vi "CurrentCollectOnly.vi"() -> ()   [LabVIEW 2018]
uses:
  <vilib>/Utility/file.llb/Write Delimited Spreadsheet (string).vi
  Drivers/Agilent 34972/Agilent 34970.lvlib
panel:
  in  "Agilent Scan Rate (Seconds)":i32=3
  in  "Start DAQ Loop":bool
  out "Collecting Agilent Data":bool
  in  "Lab?":string="Washer HCC"
  in  "?":enum32{"Main", "Extra", "Debug"}(tab)
  in  "34972-1":refnum<visa-resource-name>="AGILENT_HCC"
  in  "error in (no error)":errorcluster
  out "error out":errorcluster
  out "Data Folder":path
  out "Current Data (for each station)":string[][](array[string])
  out "XY Graph":T1(graph)
  in  "X-Axis":string(combo)
  in  "Y-Axis-1":string(combo)
  in  "Y-Axis-2":string(combo)
  out "Agilent Channels DAQ":string
  out "read buffer":string
  in  "Status Output Locations":path[](array[path])
  in  "Connected Board ID's (Newfi)":string[](array[string])
  in  "Total Array":string[][](array[string])
  out "Main Loop Rate":dbl format="%0.2f"
  out "Station IDs":string[](array[string])=["2M1", "2M2", "2M3", "2M4", "2M5", "2M6", "2M7", "2M8", "2M9", "2M10", "2M11", "2M12", "2M13", "2M14", "2M15", "2M16", "2M17", "2M18", "2M19", "2M20", "N/A", "N/A", "N/A", "N/A"]
  in  "file path (use dialog)":path
  out "DAQ Loop":string[](array[string])
  in  "Debug":bool
  in  "Timer":dbl format="%<%H:%M:%S>t"
  in  "QUIT":bool
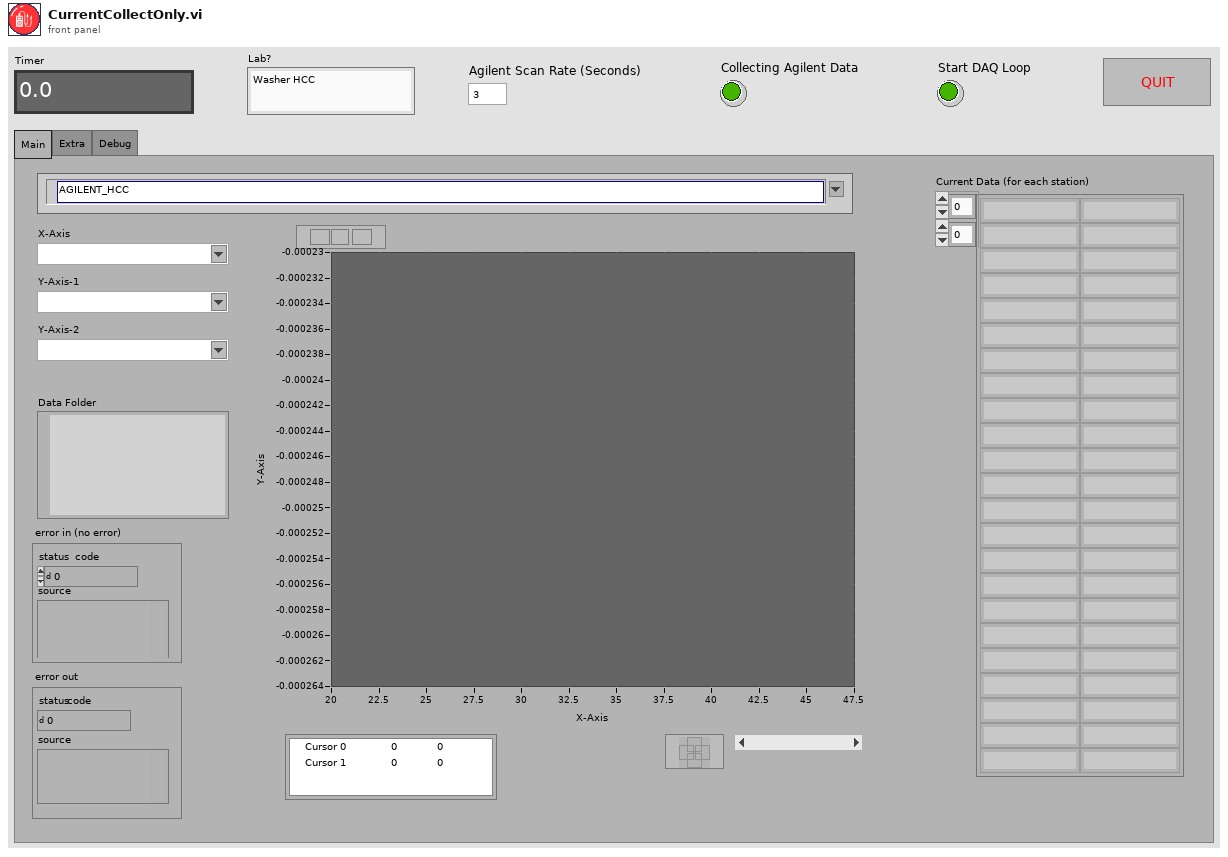
[diagram p1: front panel]
types:
  T1 = cluster{"Time Array Output":dbl[], "Data Array Output":dbl[]}[]
  T2 = cluster{"34972-1":refnum<visa-resource-name>, "Agilent Scan Rate (Seconds)":i32, "Current":dbl[], "Voltage":dbl[], "Agilent Channels DAQ":string, "file path (use dialog)":path, "Timer":dbl, "Total Array":string[][], "Station IDs":string[], "Connected Board ID's (Newfi)":string[], "Status Output Locations":path[], "Lab?":string, "Plot Array":dbl[][]}
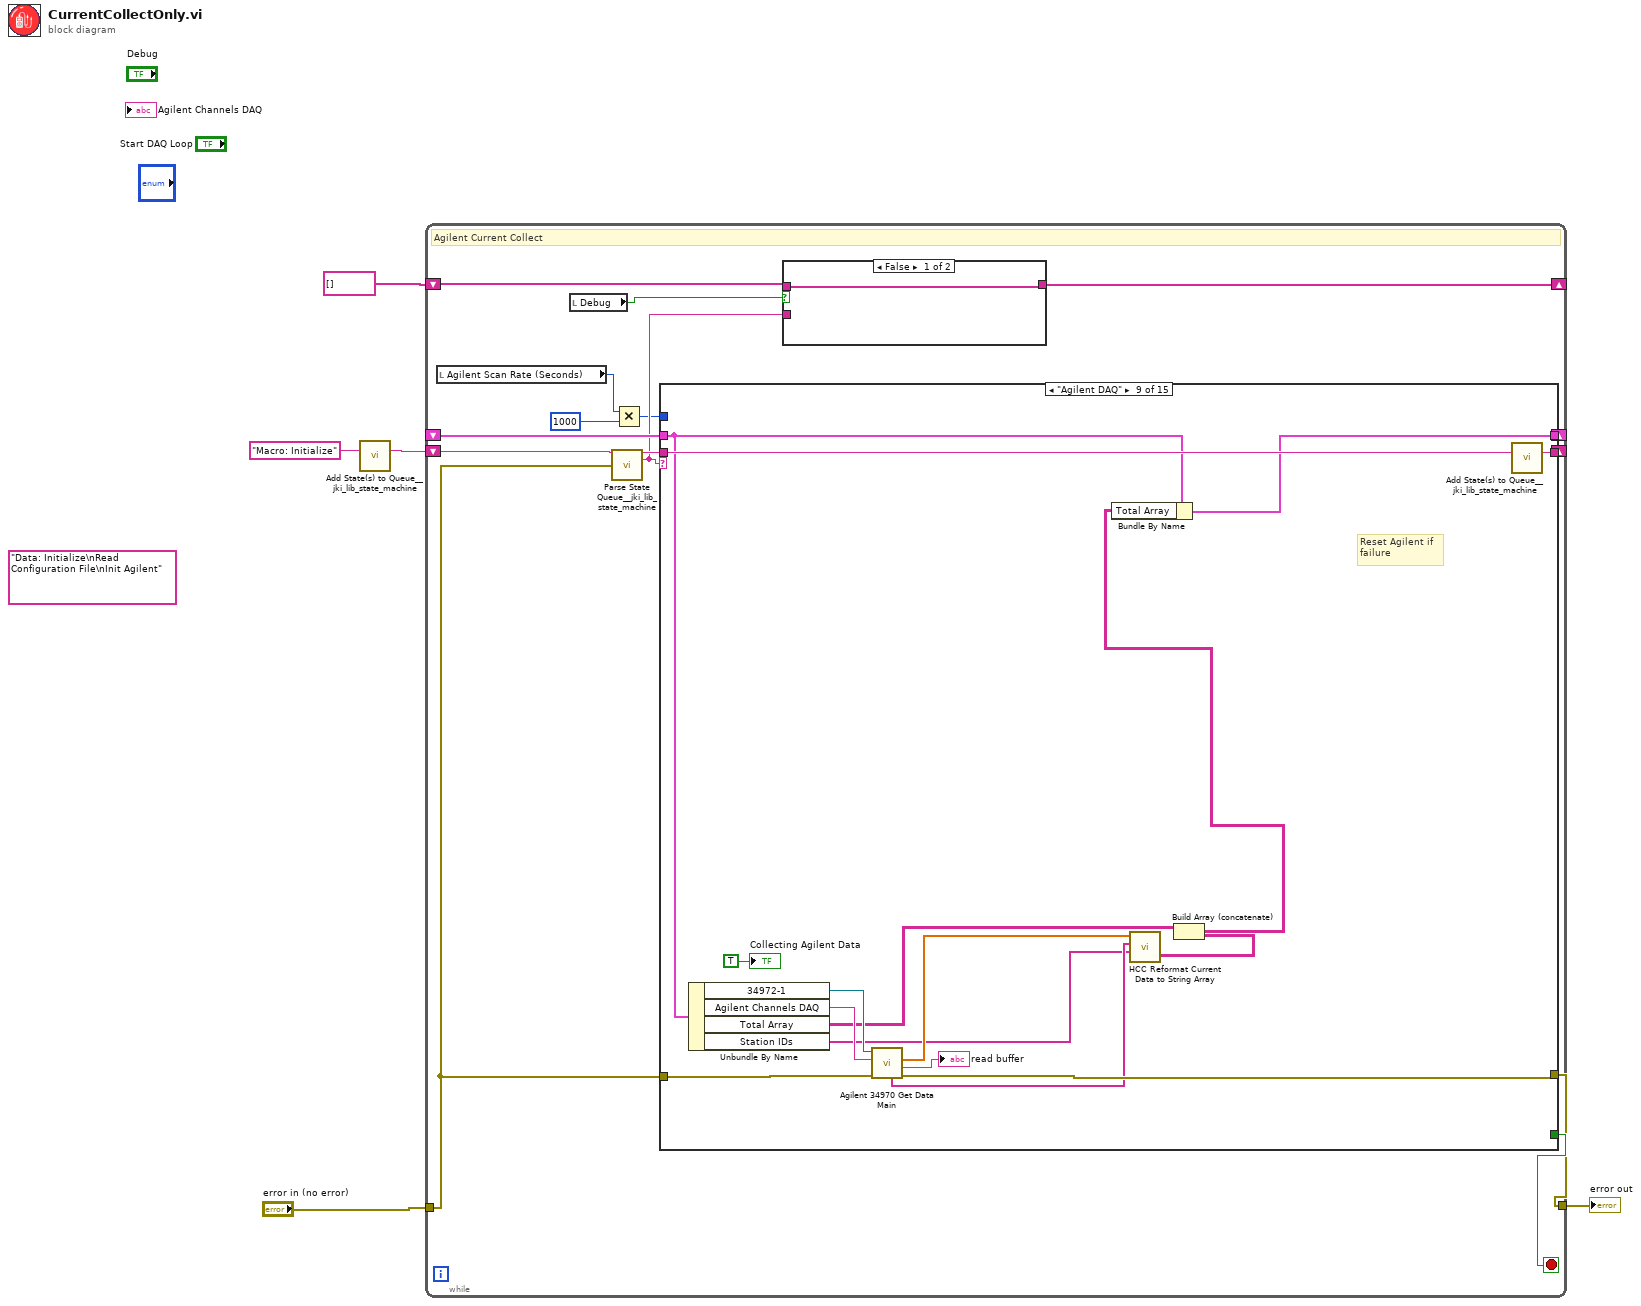
[diagram p0: block diagram]
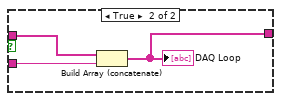
[diagram p2: hidden frame]
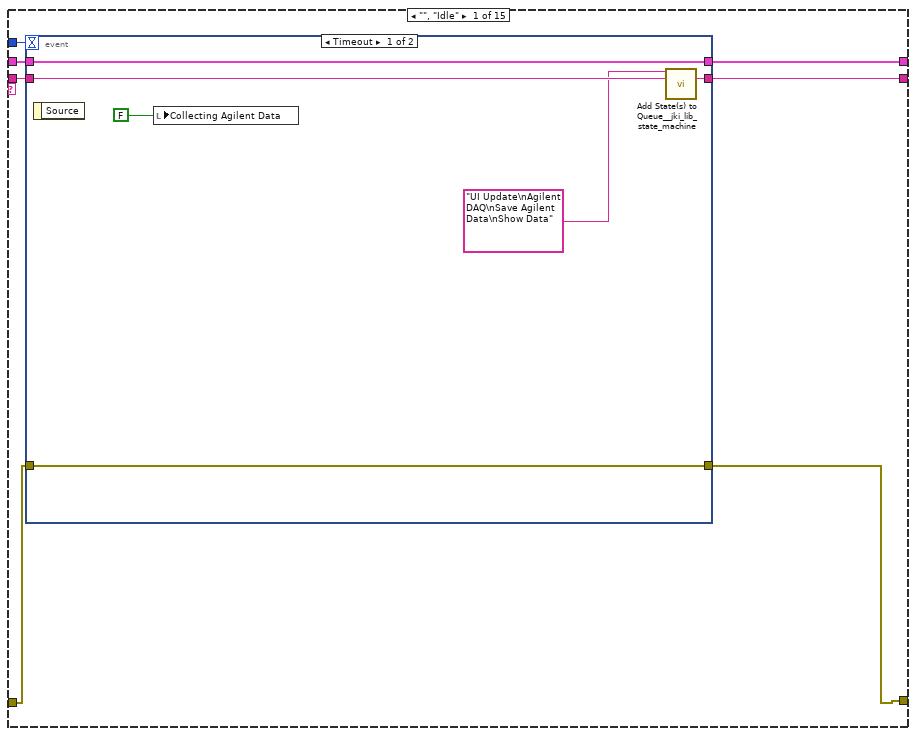
[diagram p3: hidden frame]
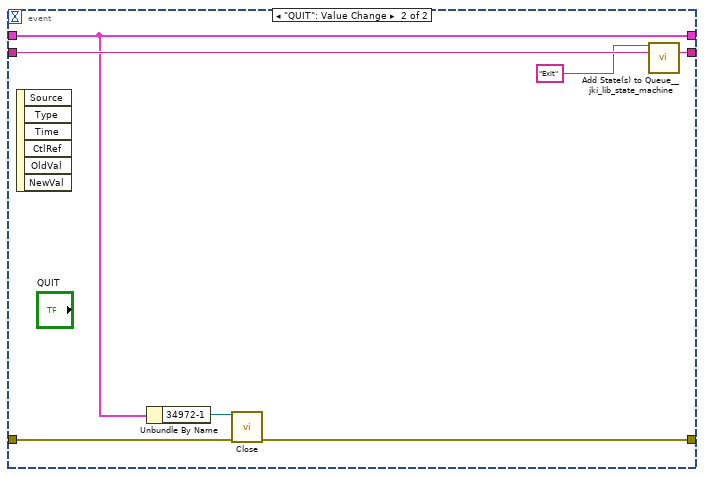
[diagram p4: hidden frame]
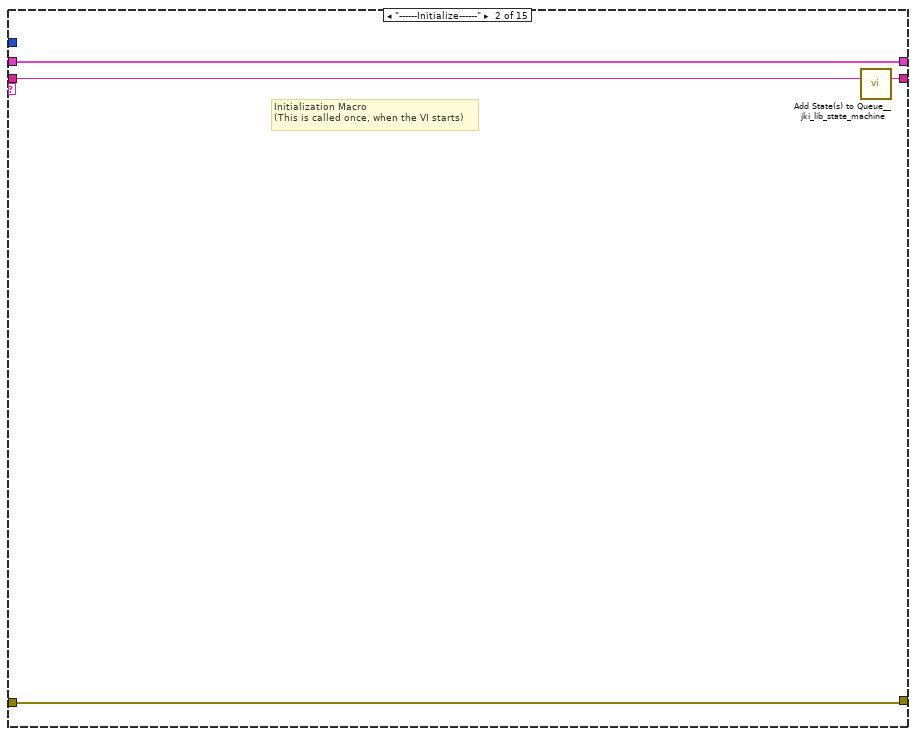
[diagram p5: hidden frame]
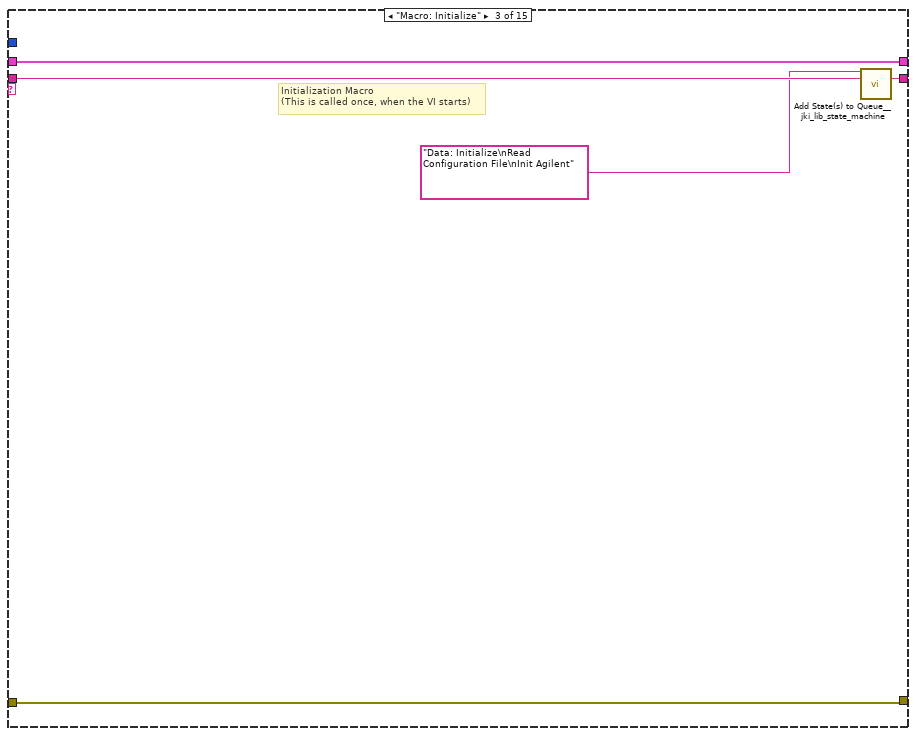
[diagram p6: hidden frame]
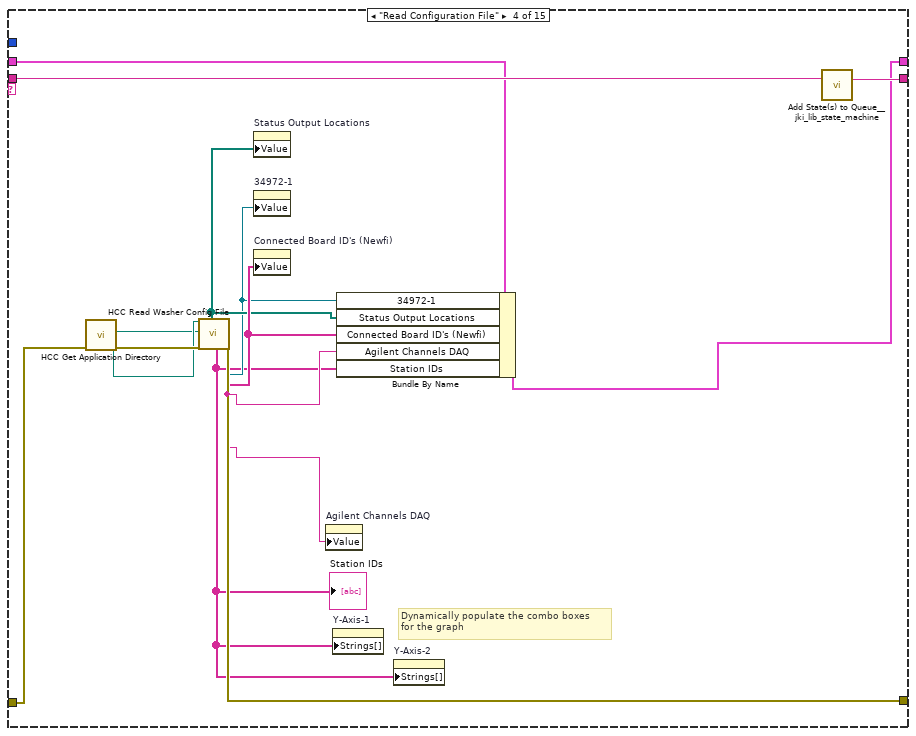
[diagram p7: hidden frame]
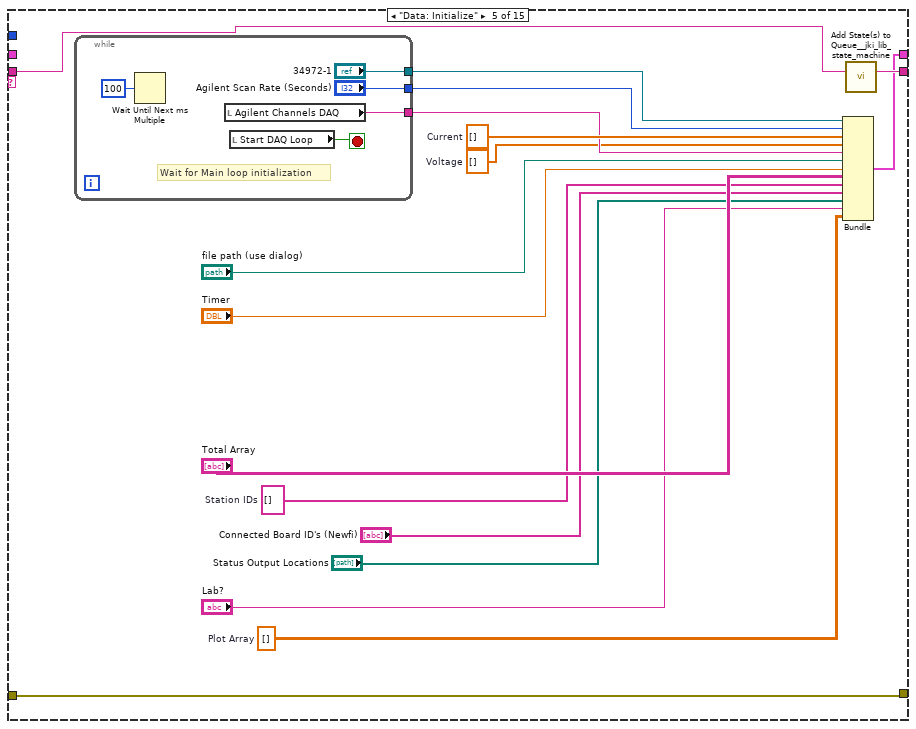
[diagram p8: hidden frame]
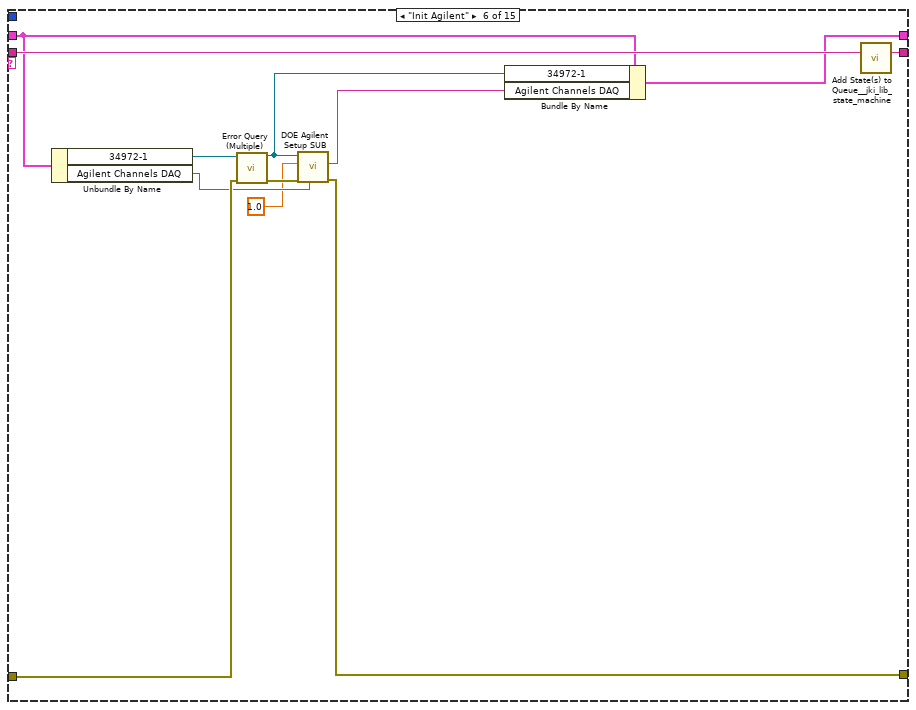
[diagram p9: hidden frame]
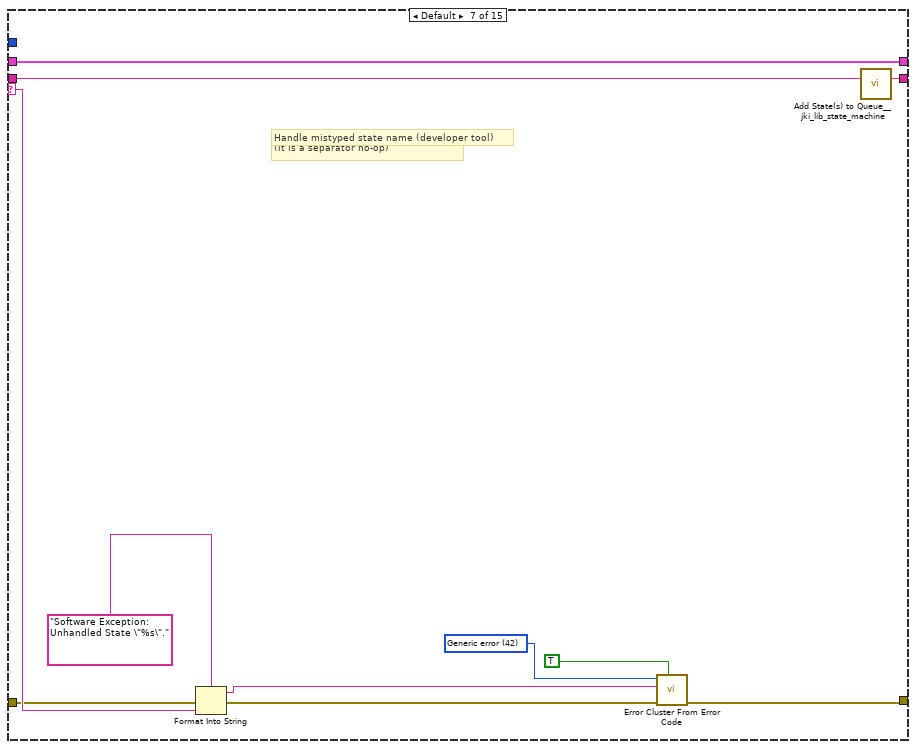
[diagram p10: hidden frame]
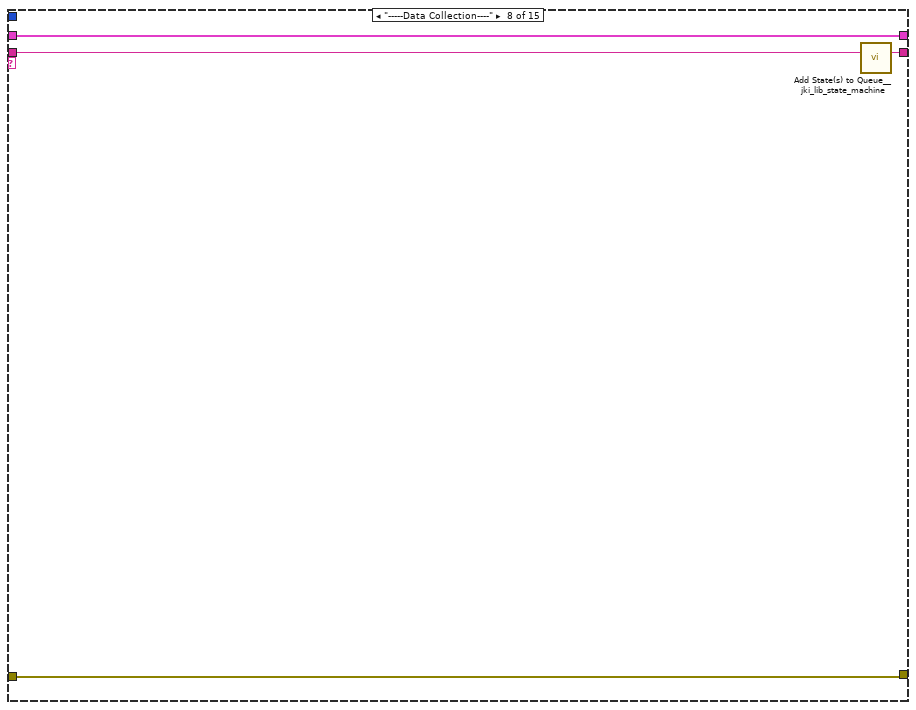
[diagram p11: hidden frame]
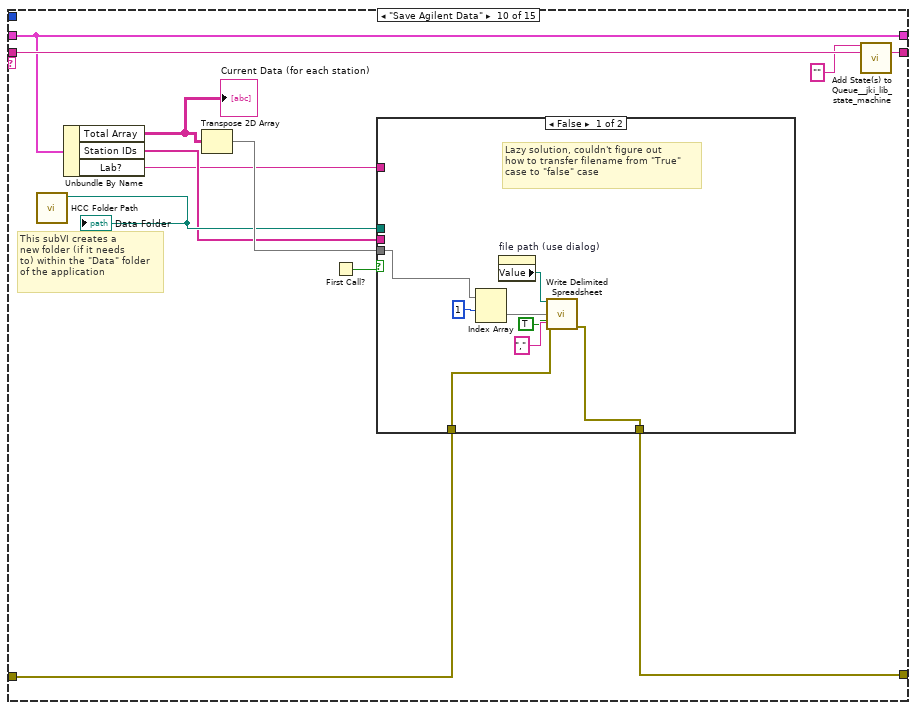
[diagram p12: hidden frame]
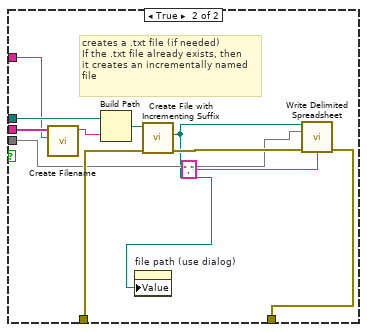
[diagram p13: hidden frame]
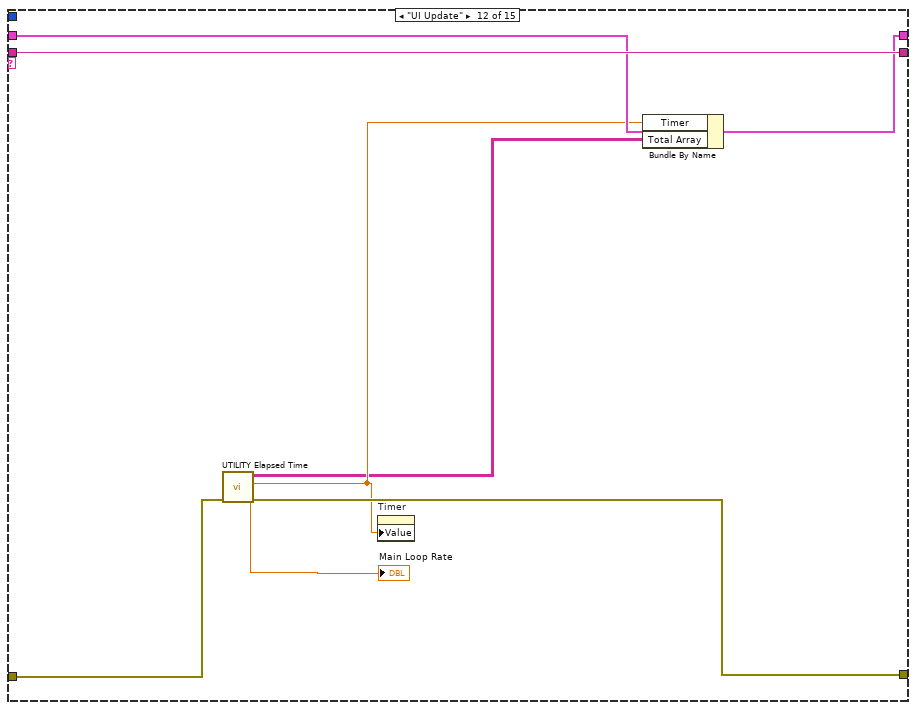
[diagram p15: hidden frame]
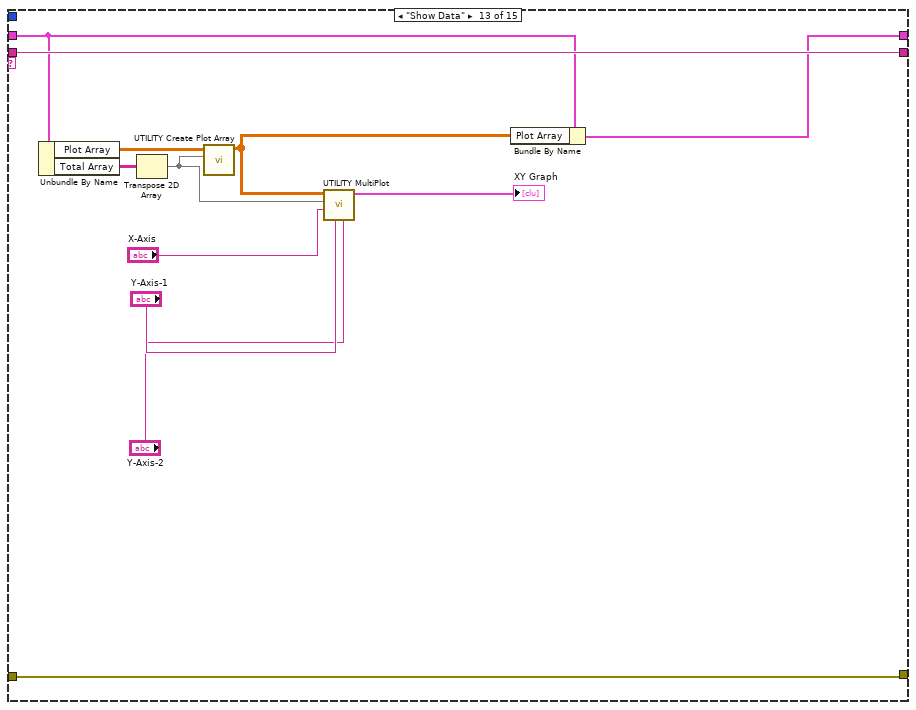
[diagram p16: hidden frame]
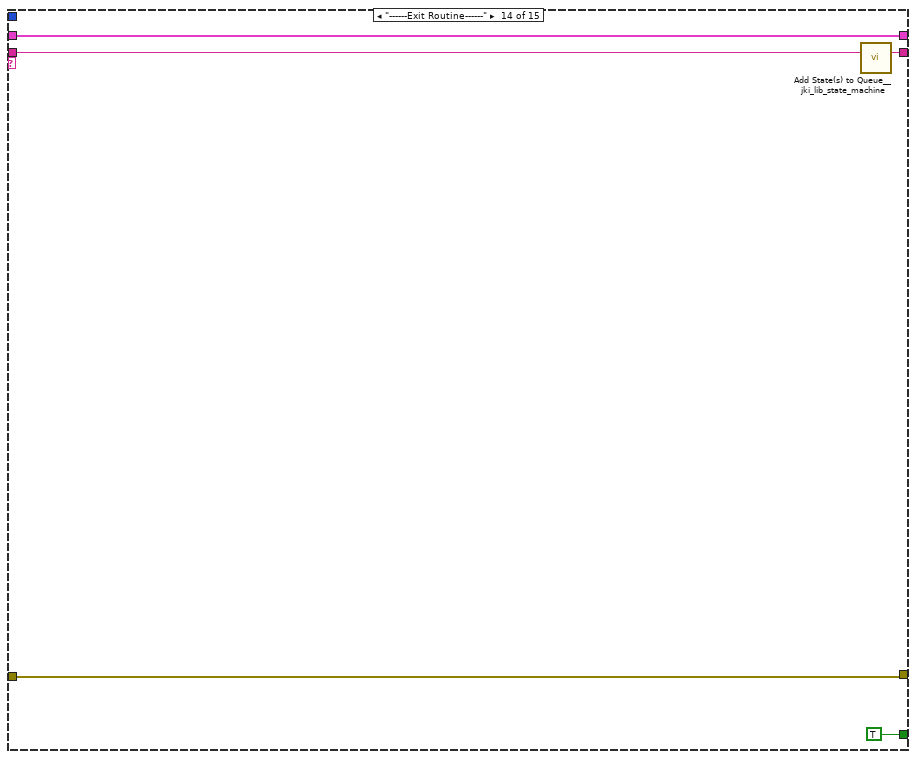
[diagram p17: hidden frame]
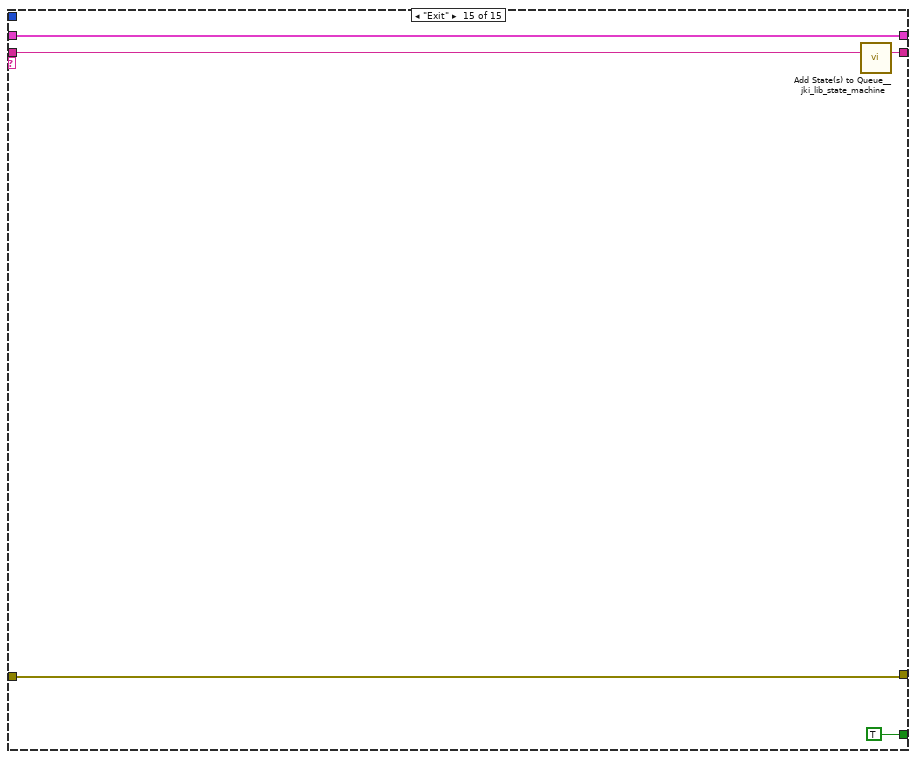
[diagram p18: hidden frame]
diagram:
  (unwired) "Data: Initialize\nRead Configuration File\nInit Agilent"
  n1 = call <vilib>:"Add State(s) to Queue__jki_lib_state_machine.vi"("State(s) in (\"\")"="Macro: Initialize") -> ("States Out"=w3:string)  [unwired: 14 in]
  n2 = while "Agilent DAQ and Save" {
    shift-right: [w6] -> _
    shift-left: _ -> [w17]
    shift-right: [w7] -> _
    shift-left: w3 -> [w19]
    tunnel: "error in (no error)" -> [w15]
    tunnel: [w16] -> w5
    shift-right: [w12] -> _
    shift-left: string[] [] -> [w14]
    stop <- w18 stop-if-true
    # "Agilent Current Collect"
    n3 = local read "Agilent Scan Rate (Seconds)"() -> (w10:i32)
    n4 = local read "Debug"() -> (w11:bool)
    n5 = call <vilib>:"Parse State Queue__jki_lib_state_machine.vi"("State Queue"=w19, "Error In (no error)"=w15) -> ("Remaining States"=w20:string, "Current State"=w13:string)  [unwired: 11 in, 1 out]
    n6 = Multiply(x=w10, y=1000) -> (x*y=w8:i32)
    n7 = case shown="\"Agilent DAQ\"" w13 {
      selector: w13 -> [_ _ _ _ _ _ w104 _ _ _ _ _ _ _ _]
      tunnel: w20 -> [w31 w48 w53 w62 w75 w101 w112 w116 w132 w144 w165 w173 w185 w191 w196]
      tunnel: w17 -> [w29 w46 w51 w61 _ w99 w110 w114 w121 w141 w166 w169 w177 w189 w194]
      tunnel: [_ _ _ _ _ _ _ _ _ _ _ _ _ TRUE TRUE] -> w18
      tunnel: w8 -> [w27 _ _ _ _ _ _ _ _ _ _ _ _ _ _]
      tunnel: w15 -> [w26 w45 w49 w67 w81 w96 w103 w113 w129 w139 w164 w174 w186 w187 w192]
      tunnel: [w25 w45 w49 w65 w81 w90 w102 w113 w125 w138 w164 w171 w186 w187 w192] -> w16
      tunnel: [w30 w47 w52 w63 w84 w100 w111 w115 w131 w143 w165 w173 w185 w190 w195] -> w7
      tunnel: [w28 w46 w51 w58 w83 w98 w110 w114 w119 w141 w166 w170 w175 w189 w194] -> w6
      frame "", "Idle" {
        n8 = event shown="[0] Timeout" {
          selector: _ -> [_ _]
          dyn-events: _ -> [_ _]
          timeout: w27 -> [_ _]
          tunnel: w31 -> [w37 w44]
          tunnel: [w36 w43] -> w30
          tunnel: w29 -> [w35 w41]
          tunnel: [w35 w41] -> w28
          tunnel: [w32 w38] -> w25
          tunnel: w26 -> [w32 w39]
          event Timeout {
            n9 = event-data() -> ()  [unwired: 1 in, 1 out]
            n10 = local write "Collecting Agilent Data"(FALSE ("Collecting Agilent Data")) -> ()
            n11 = call <vilib>:"Add State(s) to Queue__jki_lib_state_machine.vi"("State(s) in Front (\"\")"="UI Update\nAgilent DAQ\nSave Agilent Data\nShow Data", "State(s) in (\"\")"=w37) -> ("States Out"=w36:string)  [unwired: 13 in]
          }
          event "QUIT": Value Change {
            n12 = event-data() -> ()  [unwired: 1 in, 6 out]
            n13 = Unbundle By Name(w41) -> ("34972-1"=w40:refnum<visa-resource-name>)
            n14 = call "Close.vi"("VISA Resource Name"=w40, "error in (no error)"=w39) -> ("error out"=w38:errorcluster)  [unwired: 13 in]
            n15 = call <vilib>:"Add State(s) to Queue__jki_lib_state_machine.vi"("State(s) in Front (\"\")"="Exit", "State(s) in (\"\")"=w44) -> ("States Out"=w43:string)  [unwired: 13 in]
          }
        }
      }
      frame "------Initialize------" {
        # "Initialization Macro\n(This is called once, when the VI starts)"
        n16 = call <vilib>:"Add State(s) to Queue__jki_lib_state_machine.vi"("State(s) in (\"\")"=w48) -> ("States Out"=w47:string)  [unwired: 14 in]
      }
      frame "Macro: Initialize" {
        # "Initialization Macro\n(This is called once, when the VI starts)"
        n17 = call <vilib>:"Add State(s) to Queue__jki_lib_state_machine.vi"("State(s) in Front (\"\")"="Data: Initialize\nRead Configuration File\nInit Agilent", "State(s) in (\"\")"=w53) -> ("States Out"=w52:string)  [unwired: 13 in]
      }
      frame "Read Configuration File" {
        # "Dynamically populate the combo boxes\nfor the graph"
        n18 = call "HCC Get Application Directory.vi"("Error In"=w67) -> ("Error Out"=w66:errorcluster, "Configuration Path out"=w57:path, "Station and Board IDs out"=w64:path)  [unwired: 5 in, 3 out]
        n19 = call "HCC Read Washer Config File.vi"("Station and Board IDs"=w64, "Configuration Path"=w57, "Error In"=w66) -> ("Status Output Locations"=w59:path[], "Station IDs"=w54:string[], "34972A_1"=w55:refnum<visa-resource-name>, "Board ID's"=w60:string[], "Agilent Channels DAQ"=w56:string, "Error Out"=w65:errorcluster)  [unwired: 8 in, 3 out]
        "Station IDs" <- w54
        n20 = property on="Status Output Locations" class="Arr (strict)"("Value"=w59) -> ()  [unwired: 2 in, 2 out]
        n21 = property on="34972-1" class="VISAName"("Value"=w55) -> ()  [unwired: 2 in, 2 out]
        n22 = property on="Connected Board ID's (Newfi)" class="Arr (strict)"("Value"=w60) -> ()  [unwired: 2 in, 2 out]
        n23 = property on="Agilent Channels DAQ" class="Str"("Value"=w56) -> ()  [unwired: 2 in, 2 out]
        n24 = property on="Y-Axis-1" class="CmbBox"("Strings[]"=w54) -> ()  [unwired: 2 in, 2 out]
        n25 = Bundle By Name(cluster=w61, "34972-1"=w55, "Status Output Locations"=w59, "Connected Board ID's (Newfi)"=w60, "Agilent Channels DAQ"=w56, "Station IDs"=w54) -> (w58:T2)
        n26 = property on="Y-Axis-2" class="CmbBox"("Strings[]"=w54) -> ()  [unwired: 2 in, 2 out]
        n27 = call <vilib>:"Add State(s) to Queue__jki_lib_state_machine.vi"("State(s) in (\"\")"=w62) -> ("States Out"=w63:string)  [unwired: 14 in]
      }
      frame "Data: Initialize" {
        w68 = dbl[][] []  # Plot Array
        w72 = string[] []  # Station IDs
        w77 = dbl[] []  # Voltage
        w82 = dbl[] []  # Current
        n28 = while {
          tunnel: ["34972-1"] -> w78
          tunnel: ["Agilent Scan Rate (Seconds)"] -> w80
          tunnel: [w85] -> w79
          stop <- w88 stop-if-true
          # "Wait for Main loop initialization"
          n29 = Wait Until Next ms Multiple(millisecond multiple=u32 100) -> ()  [unwired: 1 out]
          n30 = local read "Agilent Channels DAQ"() -> (w85:string)
          n31 = local read "Start DAQ Loop"() -> (w88:bool)
        }
        n32 = Bundle("34972-1"=w78, "Agilent Scan Rate (Seconds)"=w80, "Current"=w82, "Voltage"=w77, "Agilent Channels DAQ"=w79, "file path (use dialog)"="file path (use dialog)", "Timer"="Timer", "Total Array"="Total Array", "Station IDs"=w72, "Connected Board ID's (Newfi)"="Connected Board ID's (Newfi)", "Status Output Locations"="Status Output Locations", "Lab?"="Lab?", "Plot Array"=w68) -> (w83:T2)  [unwired: 1 in]
        n33 = call <vilib>:"Add State(s) to Queue__jki_lib_state_machine.vi"("State(s) in (\"\")"=w75) -> ("States Out"=w84:string)  [unwired: 14 in]
      }
      frame "Init Agilent" {
        n34 = Unbundle By Name(w99) -> ("34972-1"=w97:refnum<visa-resource-name>, "Agilent Channels DAQ"=w94:string)
        n35 = call "Error Query (Multiple).vi"("VISA Resource Name"=w97, "error in (no error)"=w96) -> ("VISA Resource Name Out"=w92:refnum<visa-resource-name>, "error out"=w95:errorcluster)  [unwired: 10 in, 2 out]
        n36 = call "DOE Agilent Setup SUB.vi"("Analog Channels-List"=w94, "error in (no error)"=w95, "Agilent Gain"=1.0, "VISA Refnum in"=w92) -> ("error out"=w90:errorcluster, "Clean Analog Scan List"=w93:string)  [unwired: 5 in, 1 out]
        n37 = Bundle By Name(cluster=w99, "34972-1"=w92, "Agilent Channels DAQ"=w93) -> (w98:T2)
        n38 = call <vilib>:"Add State(s) to Queue__jki_lib_state_machine.vi"("State(s) in (\"\")"=w101) -> ("States Out"=w100:string)  [unwired: 14 in]
      }
      frame Default {
        w106 = 42 items=["No error", "Argument error", "Memory is full", "Out of zone", "End of file", "File already open", "Generic file I/O error", "File not found", "File permission error", "Disk is full", "Duplicate path", "Too many files open", "System feature not enabled", "Resource file not found", "Cannot add resource", "Resource not found", "Image not found", "Image memory error", "Pen does not exist", "Config type invalid", "Config token not found", "Config parse error", "Config memory error", "Bad external code format", "Bad external code offset", "External code not present", "Null window", "Destroy window error", "Null menu", "Print aborted", "Bad print record", "Print driver error", "Windows error during printing", "Memory error during printing", "Print dialog error", "Generic print error", "Invalid device refnum", "Device not found", "Device parameter error", "Device unit error", "Cannot open device", "Device call aborted", "Generic error", "Cancelled by user", "Object ID too low", "Object ID too high", "Object not in heap", "Unknown heap", "Unknown object (invalid DefProc)", "Unknown object (DefProc not in table)", "Message out of range", "Invalid (null) method", "Unknown message", "Manager call not supported", "Bad address", "Network operation in progress", "Network operation timed out", "Connection is busy", "Network attribute not supported", "Network error", "Address in use", "System out of memory", "Connection aborted", "Connection refused", "Not connected", "Already connected", "Connection closed", "Initialization error (interapplication manager)", "Bad occurrence", "Wait on unbound occurrence handler", "Occurrence queue overflow", "Datalog type conflict", "Unused", "Unrecognized type (interapplication manager)", "Memory corrupt", "Failed to make temporary DLL", "Old CIN version", "Drag socket not found", "Failed to load drop-object", "Failed to register OLE object", "Failed to release OLE object", "Format specifier type mismatch", "Unknown format specifier", "Too few format specifiers", "Too many format specifiers", "Scan failed", "Newer CIN version", "Error converting to variant", "Runtime menu error", "Password tampered", "Variant attribute not found", "Incompatible variant data type", "Event data is not available", "Event Store is not present", "Occurrence is not found", "Event Queue is not created", "Event info is not available", "Refnum passed is NULL", "Error retrieving Class GUID", "Error retrieving CoClass GUID", "Error retrieving TypeLib GUID.", "Bad built application magic bytes.", "Specific driver is different from the specific driver associated with the Logical Name.", "There is no session opened to the class driver.", "Max Error", "MAX - Error with config objects", "MAX - Error loading configuration", "MAX - Group not supported"]
        # "Handle mistyped state name (developer tool)"
        # "Do not put any code in this frame.\n(it is a separator no-op)"
        n39 = Format Into String(format string="Software Exception: Unhandled State \"%s\"." ("message"), error in=w103, w104) -> (resulting string=w107:string, error out=w108:errorcluster)  [unwired: 1 in]
        n40 = call <vilib>:"Error Cluster From Error Code.vi"("show call chain? (False)"=TRUE, "error in (no error)"=w108, "error message (\"\")"=w107, "error code (0)"=w106) -> ("error out"=w102:errorcluster)  [unwired: 5 in]
        n41 = call <vilib>:"Add State(s) to Queue__jki_lib_state_machine.vi"("State(s) in (\"\")"=w112) -> ("States Out"=w111:string)  [unwired: 14 in]
      }
      frame "-----Data Collection----" {
        n42 = call <vilib>:"Add State(s) to Queue__jki_lib_state_machine.vi"("State(s) in (\"\")"=w116) -> ("States Out"=w115:string)  [unwired: 14 in]
      }
      frame "Agilent DAQ" {
        # "Reset Agilent if \nfailure"
        n43 = Unbundle By Name(w121) -> ("34972-1"=w128:refnum<visa-resource-name>, "Agilent Channels DAQ"=w127:string, "Total Array"=w122:string[][], "Station IDs"=w118:string[])
        n44 = call "Agilent 34970 Get Data Main.vi"("error in (no error)"=w129, "Analog Channels-List"=w127, "VISA Refnum in"=w128) -> ("error out"=w125:errorcluster, "read buffer"=→"read buffer":string, "Sorted Data"=w124:dbl[], "Names"=w123:string[])  [unwired: 3 in, 2 out]
        n45 = call "HCC Reformat Current Data to String Array.vi"("Station IDs"=w118, "Names"=w123, "Sorted Data"=w124) -> ("Current Array"=w117:string[][])  [unwired: 8 in]
        n46 = Build Array (concatenate)(w122, w117) -> (w120:string[][])
        n47 = Bundle By Name(cluster=w121, "Total Array"=w120) -> (w119:T2)
        n48 = call <vilib>:"Add State(s) to Queue__jki_lib_state_machine.vi"("State(s) in (\"\")"=w132) -> ("States Out"=w131:string)  [unwired: 14 in]
        "Collecting Agilent Data" <- TRUE
      }
      frame "Save Agilent Data" {
        # "This subVI creates a \nnew folder (if it needs\nto) within the \"Data\" folder\nof the application"
        n49 = call "HCC Folder Path.vi"() -> ("appended path"=w135:path)  [unwired: 11 in]
        "Data Folder" <- w135
        n50 = Unbundle By Name(w141) -> ("Total Array"=w137:string[][], "Station IDs"=w134:string[], "Lab?"=w133:string)
        "Current Data (for each station)" <- w137
        n51 = Transpose 2D Array(2D array=w137) -> (transposed array=w136:string[][])
        n52 = First Call?() -> (First Call?: T/F=w140:bool)
        n53 = case shown="False" w140 {
          tunnel: w139 -> [w150 w161]
          tunnel: [w149 w162] -> w138
          tunnel: w136 -> [w147 w159]
          tunnel: w135 -> [_ w158]
          tunnel: w134 -> [_ w155]
          tunnel: w133 -> [_ w154]
          frame False {
            # "Lazy solution, couldn't figure out\nhow to transfer filename from \"True\"\ncase to \"false\" case"
            n54 = Index Array(array=w147, index (row)=1) -> (element=w146:string[])  [unwired: 1 in]
            n55 = property on="file path (use dialog)" class="Path"() -> ("Value"=w145:path)  [unwired: 2 in, 2 out]
            n56 = call-poly <vilib>:"Write Delimited Spreadsheet.vi"("file path (dialog if empty)"=w145, "1D data"=w146, "append to file? (new file:F)"=TRUE, "error in (no error)"=w150, "delimiter (\\t)"="," ("delimiter (\\t)")) -> ("error out"=w149:errorcluster)  [unwired: 9 in, 1 out]
          }
          frame True {
            # "creates a .txt file (if needed)\nIf the .txt file already exists, then\nit creates an incrementally named\nfile"
            n57 = call "Create Filename.vi"("lab?"=w154, "Array"=w155) -> ("Filename Output"=w156:string)  [unwired: 9 in]
            n58 = Build Path(base path=w158, name or relative path=w156) -> (appended path=w157:path)
            n59 = call <vilib>:"Create File with Incrementing Suffix.vi"("error in (no error)"=w161, "file path"=w157) -> ("error out"=w160:errorcluster, "actual path"=w153:path)  [unwired: 7 in, 1 out]
            n60 = property on="file path (use dialog)" class="Path"("Value"=w153) -> ()  [unwired: 2 in, 2 out]
            n61 = call-poly <vilib>:"Write Delimited Spreadsheet.vi"("file path (dialog if empty)"=w153, "2D data"=w159, "error in (no error)"=w160, "delimiter (\\t)"="," ("delimiter (\\t)")) -> ("error out"=w162:errorcluster)  [unwired: 10 in, 1 out]
          }
        }
        n62 = call <vilib>:"Add State(s) to Queue__jki_lib_state_machine.vi"("State(s) in Front (\"\")"="" ("State(s) in Front (\"\")"), "State(s) in (\"\")"=w144) -> ("States Out"=w143:string)  [unwired: 13 in]
      }
      frame "---------UI------------" {
      }
      frame "UI Update" {
        n63 = call "UTILITY Elapsed Time.vi"("error in (no error)"=w174) -> ("error out"=w171:errorcluster, "Main Loop Rate"=→"Main Loop Rate":dbl, "Elapsed Time"=w168:dbl, "Total Array"=w167:string[][])  [unwired: 6 in, 1 out]
        n64 = property on="Timer" class="DigNum (strict)"("Value"=w168) -> ()  [unwired: 2 in, 2 out]
        n65 = Bundle By Name(cluster=w169, "Timer"=w168, "Total Array"=w167) -> (w170:T2)
      }
      frame "Show Data" {
        n66 = Unbundle By Name(w177) -> ("Plot Array"=w184:dbl[][], "Total Array"=w183:string[][])
        n67 = Transpose 2D Array(2D array=w183) -> (transposed array=w182:string[][])
        n68 = call "UTILITY Create Plot Array.vi"("Save Data"=w182, "Plot Array in"=w184) -> ("Plot Array out"=w176:dbl[][])  [unwired: 8 in, 1 out]
        n69 = call "UTILITY MultiPlot.vi"("Y-Axis-2"="Y-Axis-2", "Y-Axis-1"="Y-Axis-1", "X-Axis"="X-Axis", "Save Data"=w182, "Plot Array"=w176) -> ("Plot Cluster"=→"XY Graph":T1)  [unwired: 5 in, 1 out]
        n70 = Bundle By Name(cluster=w177, "Plot Array"=w176) -> (w175:T2)
      }
      frame "------Exit Routine------" {
        n71 = call <vilib>:"Add State(s) to Queue__jki_lib_state_machine.vi"("State(s) in (\"\")"=w191) -> ("States Out"=w190:string)  [unwired: 14 in]
      }
      frame "Exit" {
        n72 = call <vilib>:"Add State(s) to Queue__jki_lib_state_machine.vi"("State(s) in (\"\")"=w196) -> ("States Out"=w195:string)  [unwired: 14 in]
      }
    }
    n73 = case shown="False" w11 {
      tunnel: w13 -> [_ w23]
      tunnel: w14 -> [w21 w24]
      tunnel: [w21 w22] -> w12
      frame False {
      }
      frame True {
        n74 = Build Array (concatenate)(w24, w23) -> (w22:string[])
        "DAQ Loop" <- w22
      }
    }
  }
  "error out" <- w5
